vi "Update.vi"(10 "Pixel Data in":u32[][](array[numeric]), 11 "Scene in":refnum<class "Scene.lvclass">) -> (2 "Pixel Data out":u32[][](array[numeric]), 3 "Scene out":refnum<class "Scene.lvclass">)   [LabVIEW 2020, in "Scene.lvclass"]
uses:
  Scene.lvclass
  Scene.lvclass/Scene.ctl
  Graphics/Libraries/Utility/Utility.lvlib
  <vilib>/ptbypt/NI_PtbyPt.lvlib
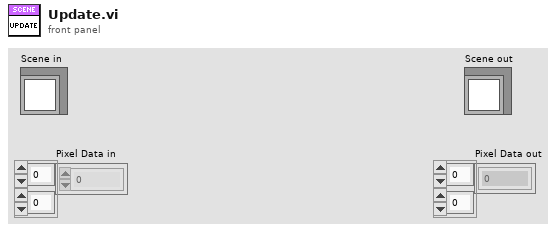
[diagram p1: front panel]
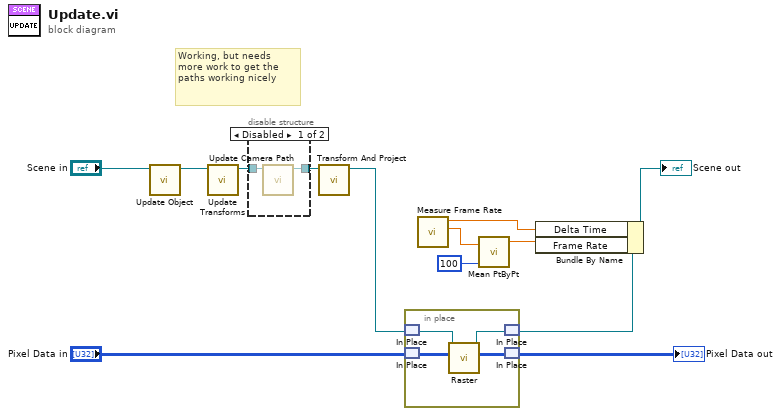
[diagram p0: block diagram]
diagram:
  # "Working, but needs more work to get the paths working nicely"
  n1 = call "Update Object.vi"("Scene in"="Scene in") -> ("Scene out"=w5:refnum<class "Scene.lvclass">)  [unwired: 10 in]
  n2 = call "Update Transforms.vi"("Scene in"=w5) -> ("Scene out"=w2:refnum<class "Scene.lvclass">)  [unwired: 10 in]
  n3 = disable-structure shown="Disabled" {
    disable-tunnel: w2 -> [w15 w16]
    disable-tunnel: [w14 w16] -> w1
    frame Disabled {
      n4 = call "Update Camera Path.vi"("Scene in"=w15) -> ("Scene out"=w14:refnum<class "Scene.lvclass">)  [unwired: 10 in]
    }
    frame Enabled {
    }
  }
  n5 = call "Transform And Project.vi"("Scene in"=w1) -> ("Scene out"=w4:refnum<class "Scene.lvclass">)  [unwired: 10 in]
  n6 = in-place {
    n7 = in-place-match #1(w4) -> (w18:refnum<class "Scene.lvclass">)
    n8 = in-place-match #2("Pixel Data in") -> (w20:u32[][])
    n9 = call "Raster.vi"("Pixel Data in"=w20, "Scene in"=w18) -> ("Pixel Data out"=w19:u32[][], "Scene out"=w17:refnum<class "Scene.lvclass">)  [unwired: 8 in]
    n10 = in-place-match #1(w17) -> (w3:refnum<class "Scene.lvclass">)
    n11 = in-place-match #2(w19) -> (→"Pixel Data out":u32[][])
  }
  n12 = call "Measure Frame Rate.vi"() -> ("Frame Rate [FPS]"=w11:dbl, "Delta Time [s]"=w7:dbl)  [unwired: 10 in]
  n13 = call <vilib>:"Mean PtByPt.vi"("x"=w11, "sample length"=100) -> ("mean"=w8:dbl)  [unwired: 2 in, 1 out]
  n14 = Bundle By Name(cluster=w3, "Delta Time"=w7, "Frame Rate"=w8) -> (→"Scene out":refnum<class "Scene.lvclass">)
